vi "Get GObj Rect.vi"(8 "错误输入（无错误）":errorcluster, 10 "Select":enum16{"TotalRect", "MasterRect"}(ring), 11 "GObj Ref In":refnum<vi>) -> (0 "错误输出":errorcluster, 1 "Bounds":T2, 2 "Position":T3, 3 "GObj Ref Out":refnum<vi>, 5 "MasterRect":T1 caption="Rect")   [LabVIEW 2012, in "CtrlRef.lvlib"]
uses:
  CtrlRef.lvlib
  <vilib>/Utility/miscctls.llb/LVPositionTypeDef.ctl
  <vilib>/Utility/miscctls.llb/LVBoundsTypeDef.ctl
  <vilib>/Utility/miscctls.llb/LVRectTypeDef.ctl
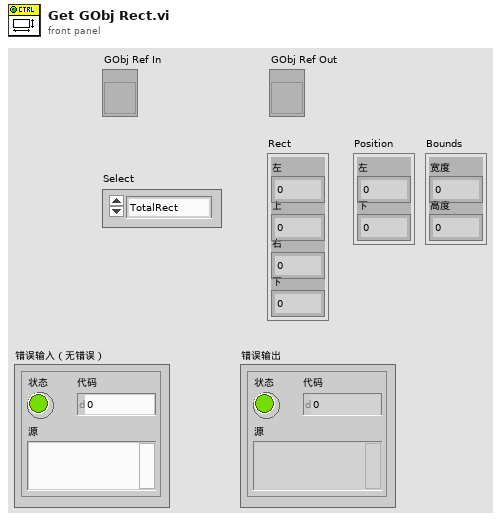
[diagram p1: front panel]
types:
  T1 = typedef "LVRectTypeDef.ctl" = cluster{"Left":i16, "Top":i16, "Right":i16, "Bottom":i16}
  T2 = typedef "LVBoundsTypeDef.ctl" = cluster{"Width":u32, "Height":u32}
  T3 = typedef "LVPositionTypeDef.ctl" = cluster{"Left":i32, "Top":i32}
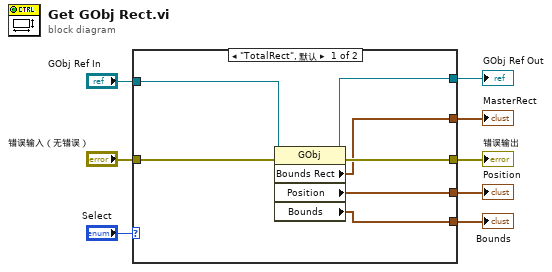
[diagram p0: block diagram]
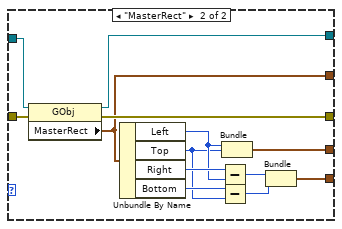
[diagram p2: hidden frame]
diagram:
  n1 = case shown="\"TotalRect\", 默认" "Select" {
    tunnel: "错误输入（无错误）" -> [w15 w27]
    tunnel: "GObj Ref In" -> [w14 w28]
    tunnel: [w13 w25] -> w1
    tunnel: [w12 w26] -> w6
    tunnel: [w11 w23] -> w5
    tunnel: [w10 w16] -> w4
    tunnel: [w9 w24] -> w3
    frame "TotalRect", Default {
      n2 = property class="GObj"(reference=w14, error in=w15) -> (reference out=w13:refnum<vi>, error out=w12:errorcluster, "Bounds Rect"=w9:T1, "Position"=w11:T3, "Bounds"=w10:T2)
    }
    frame "MasterRect" {
      n3 = property class="GObj"(reference=w28, error in=w27) -> (reference out=w25:refnum<vi>, error out=w26:errorcluster, "MasterRect"=w24:T1)
      n4 = Unbundle By Name(w24) -> ("Left"=w21:i16, "Top"=w19:i16, "Right"=w22:i16, "Bottom"=w20:i16)
      n5 = Subtract(x=w22, y=w21) -> (x-y=w17:i16)
      n6 = Subtract(x=w20, y=w19) -> (x-y=w18:i16)
      n7 = Bundle("Left"=w21, "Top"=w19) -> (w23:cluster{"Left":i16, "Top":i16})  [unwired: 1 in]
      n8 = Bundle(w17, w18) -> (w16:cluster{i16, i16})  [unwired: 1 in]
    }
  }
  "错误输出" <- w6
  "Position" <- w5
  "Bounds" <- w4
  "MasterRect" <- w3
  "GObj Ref Out" <- w1
